vi "Calculate Distances with set.vi"(8 "error in (no error)":errorcluster, 11 "Grassfire in":refnum<class "Grassfire.lvclass">) -> (0 "error out":errorcluster, 3 "Grassfire out":refnum<class "Grassfire.lvclass">)   [LabVIEW 2019, in "Grassfire.lvclass"]
uses:
  Grassfire.lvclass
  Address/Address.lvclass
  Grassfire.lvclass/Grassfire.ctl
  Node/Node.lvclass/Node.ctl
  Node/Node.lvclass
panel:
  out "Total ms":u32
  out "Iteration ms":u32
  out "i":i32
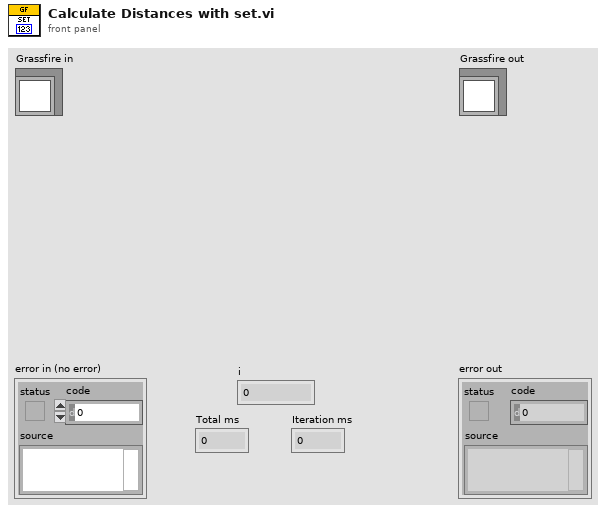
[diagram p1: front panel]
types:
  T1 = map{refnum<class "Address.lvclass">, refnum<class "Node.lvclass">}
  T2 = cluster{"Address":refnum<class "Address.lvclass">, "Step":i32}
  T3 = typedef "Shared.lvlib/Node Type--enum.ctl" = enum16{"Empty", "Blocked", "Start", "End", "Path"}
  T4 = cluster{"2D Array Index":refnum<class "Address.lvclass">, i32}
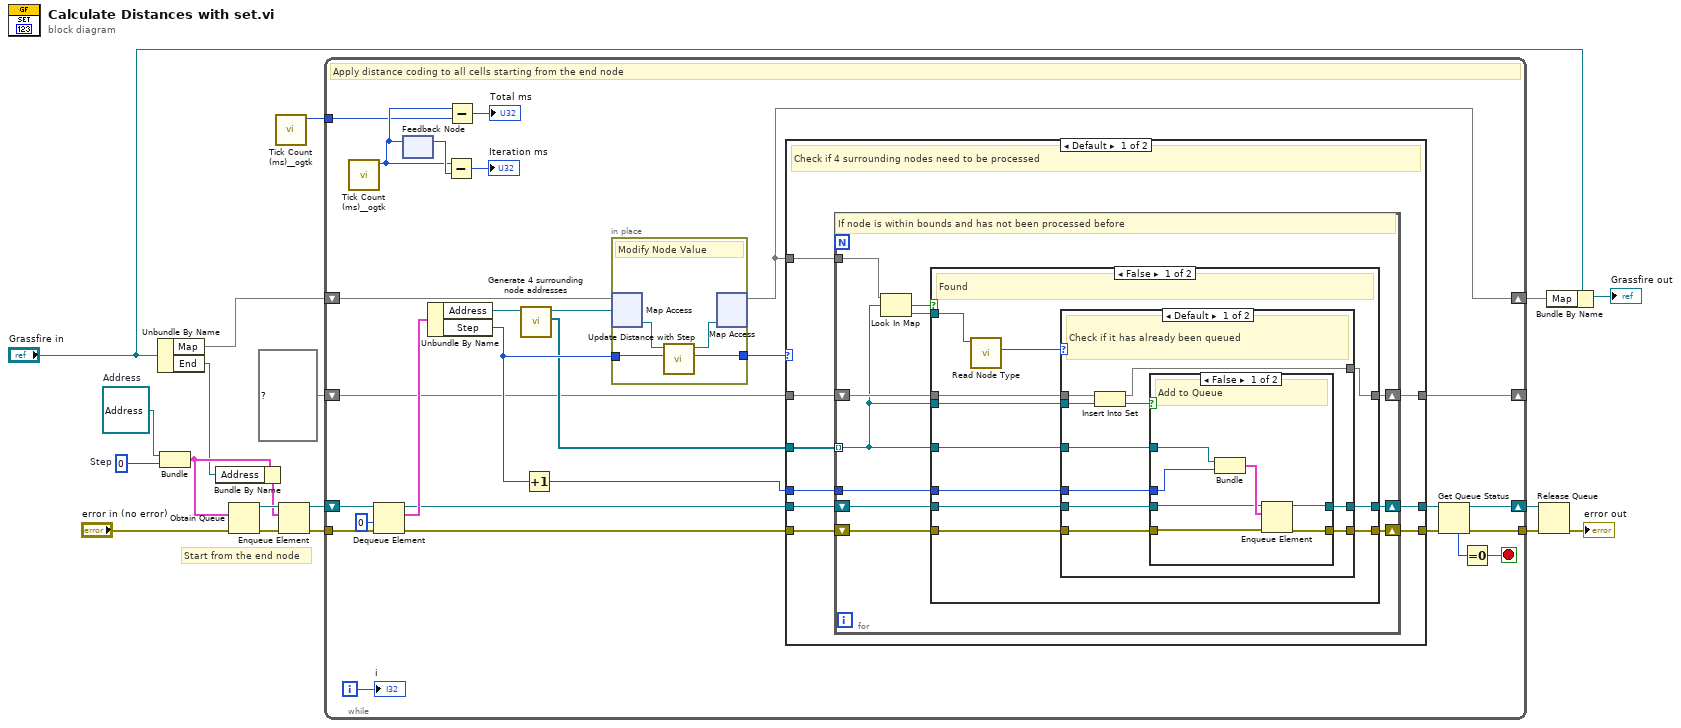
[diagram p0: block diagram]
diagram:
  w3 = refnum<class "Address.lvclass"> refnum  # Address
  w18 = 0  # Step
  # "Start from the end node"
  n1 = Unbundle By Name("Grassfire in") -> ("Map"=w13:T1, "End"=w15:refnum<class "Address.lvclass">)
  n2 = Bundle("Address"=w3, "Step"=w18) -> (w17:T2)  [unwired: 1 in]
  n3 = Bundle By Name(cluster=w17, "Address"=w15) -> (w16:T2)
  n4 = Obtain Queue(element data type=w17, error in (no error)="error in (no error)") -> (queue out=w19:refnum<queue>, error out=w10:errorcluster)  [unwired: 3 in, 1 out]
  n5 = call <userlib>:"Tick Count (ms)__ogtk.vi"() -> ("millisecond timer value"=w1:u32)  [unwired: 10 in, 1 out]
  n6 = Enqueue Element(queue=w19, element=w16, error in (no error)=w10) -> (queue out=w11:refnum<queue>, error out=w12:errorcluster)  [unwired: 1 in, 1 out]
  n7 = while {
    shift-right: [w33] -> w7
    shift-left: w13 -> [w37]
    shift-right: [w41] -> w5
    shift-left: w11 -> [w45]
    tunnel: w12 -> [w43]
    tunnel: [w42] -> w6
    shift-right: [w27] -> _
    shift-left: set{refnum<class "Address.lvclass">} {} ("set") -> [w28]
    tunnel: w1 -> [w21]
    i -> [w47]
    stop <- w40 stop-if-true
    # "Apply distance coding to all cells starting from the end node"
    n8 = call <userlib>:"Tick Count (ms)__ogtk.vi"() -> ("millisecond timer value"=w22:u32)  [unwired: 10 in, 1 out]
    n9 = Dequeue Element(queue=w45, timeout in ms (-1)=0, error in (no error)=w43) -> (queue out=w31:refnum<queue>, element=w44:T2, error out=w30:errorcluster)  [unwired: 1 out]
    n10 = feedback-in #1(w22) -> ()
    n11 = feedback #1() -> (w24:u32)  [unwired: 1 in]
    n12 = Unbundle By Name(w44) -> ("Address"=w38:refnum<class "Address.lvclass">, "Step"=w35:i32)
    n13 = Subtract(x=w22, y=w24) -> (x-y=→"Iteration ms":u32)
    n14 = Subtract(x=w22, y=w21) -> (x-y=→"Total ms":u32)
    n15 = call "Generate 4 surrounding node addresses.vi"("2D Array in"=w38) -> ("4 Surrounding Nodes"=w29:refnum<class "Address.lvclass">[], "2D Array out"=w36:refnum<class "Address.lvclass">)  [unwired: 7 in, 2 out]
    n16 = Increment(x=w35) -> (x+1=w32:i32)
    n17 = in-place {
      in-place-border: w35 -> [w108]
      in-place-border: [w107] -> w34
      # "Modify Node Value"
      n18 = in-place-map #2(w37, w36) -> (w110:refnum<class "Node.lvclass">)  [unwired: 1 in, 1 out]
      n19 = call "Update Distance with Step.vi"("Step"=w108, "Picture Ring in"=w110) -> ("Type"=w107:T3, "Picture Ring out"=w109:refnum<class "Node.lvclass">)  [unwired: 7 in, 1 out]
      n20 = in-place-map #2(w109) -> (w33:T1)  [unwired: 1 in, 2 out]
    }
    n21 = case shown="Default" w34 {
      tunnel: [w55 w106] -> w26
      tunnel: w29 -> [w54 _]
      tunnel: w31 -> [w56 w106]
      tunnel: w30 -> [w53 w105]
      tunnel: [w52 w105] -> w25
      tunnel: w33 -> [w48 _]
      tunnel: w28 -> [w51 w104]
      tunnel: w32 -> [w50 _]
      tunnel: [w49 w104] -> w27
      frame Default {
        # "Check if 4 surrounding nodes need to be processed"
        n22 = for {
          tunnel: w54 -> [w63] mode=indexing
          shift-right: [w61] -> w55
          shift-left: w56 -> [w60]
          shift-right: [w59] -> w52
          shift-left: w53 -> [w58]
          tunnel: w50 -> [w62]
          shift-right: [w64] -> w49
          shift-left: w51 -> [w65]
          tunnel: w48 -> [w57]
          # "If node is within bounds and has not been processed before"
          n23 = Look In Map(map=w57, key=w63) -> (key not found?=w66:bool, value=w67:refnum<class "Node.lvclass">)  [unwired: 1 in]
          n24 = case shown="False" w66 {
            tunnel: w67 -> [w69 _]
            tunnel: w65 -> [w78 w103]
            tunnel: [w77 w103] -> w64
            tunnel: w63 -> [w76 _]
            tunnel: w63 -> [w75 _]
            tunnel: w62 -> [w74 _]
            tunnel: [w73 w102] -> w61
            tunnel: w60 -> [w72 w102]
            tunnel: [w71 w101] -> w59
            tunnel: w58 -> [w70 w101]
            frame False {
              # "Found"
              n25 = call "Read Node Type.vi"("Picture Ring in"=w69) -> ("Type"=w68:T3)  [unwired: 8 in, 2 out]
              n26 = case shown="Default" w68 {
                tunnel: w78 -> [w88 w100]
                tunnel: [w86 w100] -> w77
                tunnel: w76 -> [w85 _]
                tunnel: w75 -> [w84 _]
                tunnel: w74 -> [w83 _]
                tunnel: [w82 w99] -> w73
                tunnel: w72 -> [w81 w99]
                tunnel: [w80 w98] -> w71
                tunnel: w70 -> [w79 w98]
                frame Default {
                  # "Check if it has already been queued"
                  n27 = Insert Into Set(10:w85, 11:w88) -> (2:w87:bool, 3:w86:set{refnum<class "Address.lvclass">})
                  n28 = case shown="False" w87 {
                    tunnel: w84 -> [w92 _]
                    tunnel: w83 -> [w91 _]
                    tunnel: [w94 w97] -> w82
                    tunnel: w81 -> [w90 w97]
                    tunnel: [w93 w96] -> w80
                    tunnel: w79 -> [w89 w96]
                    frame False {
                      # "Add to Queue"
                      n29 = Bundle("2D Array Index"=w92, w91) -> (w95:T4)  [unwired: 1 in]
                      n30 = Enqueue Element(queue=w90, element=w95, error in (no error)=w89) -> (queue out=w94:refnum<queue>, error out=w93:errorcluster)  [unwired: 1 in, 1 out]
                    }
                    frame True {
                      # "Don't Queue"
                    }
                  }
                }
                frame "Blocked" {
                  # "Don't Process"
                }
              }
            }
            frame True {
              # "Not Found"
            }
          }
        }
      }
      frame "Blocked" {
        # "Current node is blocked No further actions"
      }
    }
    n31 = Get Queue Status(queue=w26, error in (no error)=w25) -> (queue out=w41:refnum<queue>, error out=w42:errorcluster, # elements in queue=w39:i32)  [unwired: 1 in, 5 out]
    n32 = Equal To 0?(x=w39) -> (x = 0?=w40:bool)
    "i" <- w47
  }
  n33 = Release Queue(queue=w5, error in (no error)=w6) -> (error out=→"error out":errorcluster)  [unwired: 1 in, 2 out]
  n34 = Bundle By Name(cluster="Grassfire in", "Map"=w7) -> (→"Grassfire out":refnum<class "Grassfire.lvclass">)
